vi "Notifier Actor.vi"(10 "Spawn":refnum<class "Spawn.lvclass">, 11 "TEMPLATE Actor in":refnum<class "TEMPLATE Actor.lvclass">) -> (0 "Error out":errorcluster, 3 "TEMPLATE Actor out":refnum<class "TEMPLATE Actor.lvclass">)   [LabVIEW 2025, in "_Template.lvlib" / "Templates.lvlib" / "TEMPLATE Actor.lvlib" / "TEMPLATE Actor.lvclass"]
uses:
  TEMPLATE Actor.lvclass
  TEMPLATE Actor.lvclass/TEMPLATE Actor.ctl
  C:/git/jettl/src/jettl Tools/_Template/Templates/TEMPLATE Actor/TEMPLATE Actor/TEMPLATE Actor.lvclass
  C:/git/jettl/src/jettl/jettl/Actor/Actor/Actor.lvclass
  C:/git/jettl/src/jettl/jettl/Stopped Msg/Stopped/Stopped.lvclass
  jettl/jettl/Actor/Actor.lvlib
  Control Refs.ctl
  jettl/jettl/Transport/Notifier/Notifier.lvlib
  jettl/jettl/Spawn/Spawn/Spawn.lvclass
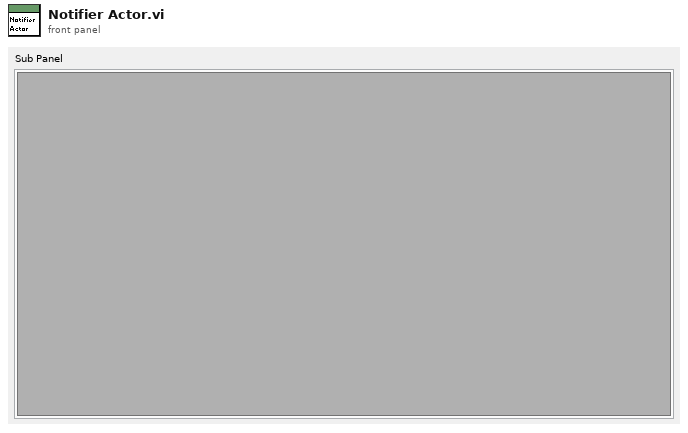
[diagram p1: front panel]
types:
  T1 = typedef "_Template.lvlib/Templates.lvlib/TEMPLATE Actor.lvlib/TEMPLATE Actor.lvclass/Control Refs.ctl" = cluster{"Sub Panel":refnum<vi>}
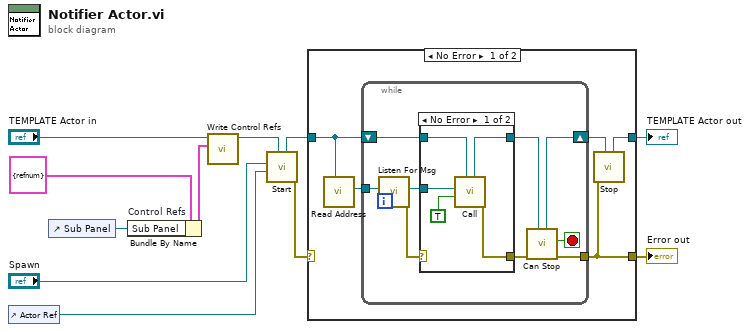
[diagram p0: block diagram]
diagram:
  n1 = control-ref of="Actor Ref"() -> (w7:refnum<vi>)
  n2 = control-ref of="Sub Panel"() -> (w1:refnum<vi>)
  n3 = Bundle By Name "Control Refs"(cluster=T1 {"Sub Panel"=refnum} ("Process Refs"), "Sub Panel"=w1) -> (w2:T1)
  n4 = call "Write Control Refs.vi"("Control Refs"=w2, "TEMPLATE Actor in"="TEMPLATE Actor in") -> ("TEMPLATE Actor out"=w3:refnum<class "TEMPLATE Actor.lvclass">)  [unwired: 9 in]
  n5 = call "Start.vi"("Actor in"=w3, "Actor Ref"=w7, "Spawn"="Spawn") -> ("Error out"=w9:errorcluster, "Actor out"=w8:refnum<class "TEMPLATE Actor.lvclass">)  [unwired: 7 in]
  n6 = case shown="No Error" w9 {
    selector: w9 -> [_ w33]
    tunnel: [w14 w34] -> w11
    tunnel: w8 -> [w13 w34]
    tunnel: [w16 w33] -> w10
    frame No Error {
      n7 = call "Read Address.vi"("Actor"=w13) -> ("Address"=w12:refnum<data-value>)  [unwired: 10 in]
      n8 = while {
        shift-right: [w23] -> w15
        shift-left: w13 -> [w21]
        tunnel: [w24] -> w16
        tunnel: w12 -> [w19]
        stop <- w22 stop-if-true
        n9 = call "Listen For Msg.vi"("Address"=w19) -> ("Error out"=w18:errorcluster, "Msg"=w17:refnum<class "Msg.lvclass">)  [unwired: 9 in]
        n10 = case shown="No Error" w18 {
          selector: w18 -> [_ w31]
          tunnel: [w30 w31] -> w25
          tunnel: w21 -> [w29 w32]
          tunnel: [w28 w32] -> w20
          tunnel: w17 -> [w27 _]
          frame No Error {
            n11 = call "Call.vi"("Actor in"=w29, "Listened To Msg"=TRUE, "Msg"=w27) -> ("Error out"=w30:errorcluster, "Actor out"=w28:refnum<class "TEMPLATE Actor.lvclass">)  [unwired: 6 in, 1 out]
          }
          frame Error {
          }
        }
        n12 = call "Can Stop.vi"("Actor in"=w20, "Error in"=w25) -> ("Error out"=w24:errorcluster, "Stop"=w22:bool, "Actor out"=w23:refnum<class "TEMPLATE Actor.lvclass">)  [unwired: 7 in]
      }
      n13 = call "Stop.vi"("Actor in"=w15, "Error in"=w16) -> ("Actor out"=w14:refnum<class "TEMPLATE Actor.lvclass">)  [unwired: 9 in]
    }
    frame Error {
    }
  }
  "TEMPLATE Actor out" <- w11
  "Error out" <- w10
